vi "countCycle.vi"() -> ()   [LabVIEW 2018]
panel:
  in  "Boolean":bool=TRUE
  out "# of Samples":i32
  out "# of Passed Samples":i32
  out "# of Failed Samples":i32
  in  "stop":bool
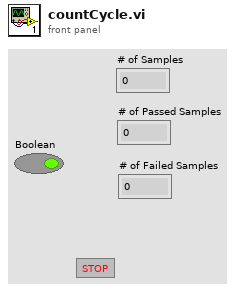
[diagram p1: front panel]
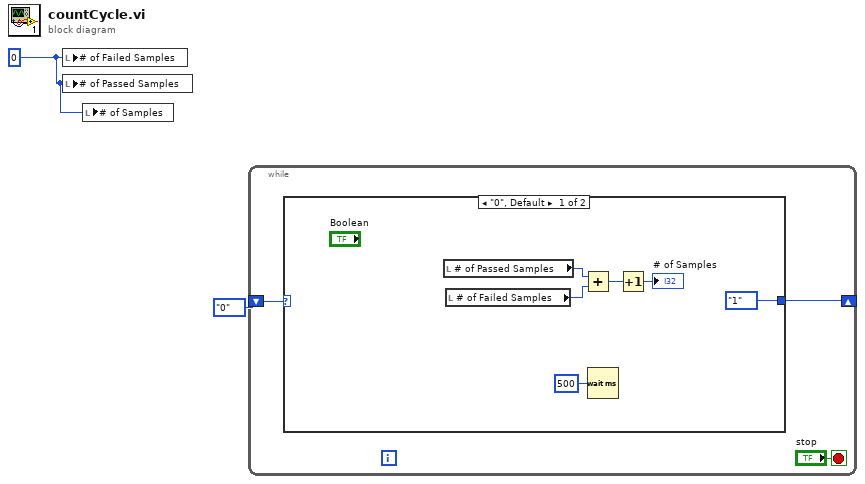
[diagram p0: block diagram]
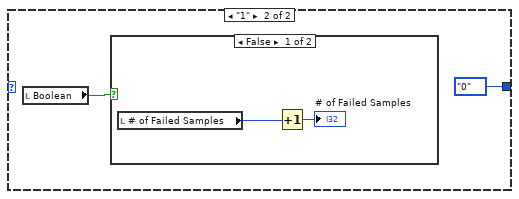
[diagram p2: hidden frame]
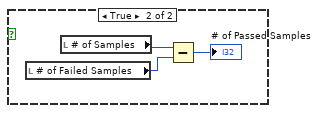
[diagram p3: hidden frame]
diagram:
  w1 = 0 ("# of Failed Samples")
  n1 = local write "# of Failed Samples"(w1) -> ()
  n2 = local write "# of Passed Samples"(w1) -> ()
  n3 = local write "# of Samples"(w1) -> ()
  n4 = while {
    shift-right: [w3] -> _
    shift-left: enum16{"0", "1"}."0" -> [w4]
    stop <- "stop" stop-if-true
    n5 = case shown="\"0\", Default" w4 {
      tunnel: [enum16{"0", "1"}."1" enum16{"0", "1"}."0"] -> w3
      frame "0", Default {
        n6 = local read "# of Passed Samples"() -> (w8:i32)
        n7 = local read "# of Failed Samples"() -> (w9:i32)
        n8 = Add(x=w8, y=w9) -> (x+y=w10:i32)
        n9 = Wait (ms)(milliseconds to wait=u32 500) -> ()  [unwired: 1 out]
        n10 = Increment(x=w10) -> (x+1=→"# of Samples":i32)
      }
      frame "1" {
        n11 = local read "Boolean"() -> (w12:bool)
        n12 = case shown="False" w12 {
          frame False {
            n13 = local read "# of Failed Samples"() -> (w14:i32)
            n14 = Increment(x=w14) -> (x+1=→"# of Failed Samples":i32)
          }
          frame True {
            n15 = local read "# of Failed Samples"() -> (w17:i32)
            n16 = local read "# of Samples"() -> (w16:i32)
            n17 = Subtract(x=w16, y=w17) -> (x-y=→"# of Passed Samples":i32)
          }
        }
      }
    }
  }
